vi "Run.vi"(8 "error in (no error)":errorcluster, 11 "App in":refnum<class "App.lvclass">) -> (0 "error out":errorcluster, 3 "App out":refnum<class "App.lvclass">)   [LabVIEW 2022 SP3, in "VMR-Deck.lvlib" / "App.lvclass"]
uses:
  App.lvclass
  App.lvclass/App.ctl
  WebServer/WebServer.lvclass
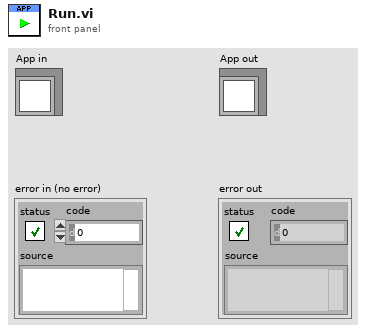
[diagram p1: front panel]
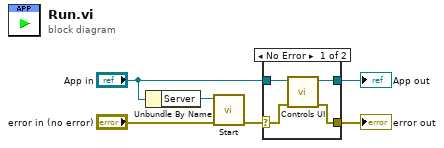
[diagram p0: block diagram]
diagram:
  n1 = Unbundle By Name("App in") -> ("Server"=w4:refnum<class "WebServer.lvclass">)
  n2 = call "Start.vi"("error in (no error)"="error in (no error)", "WebServer in"=w4) -> ("error out"=w2:errorcluster)  [unwired: 8 in, 1 out]
  n3 = case shown="No Error" w2 {
    selector: w2 -> [w8 w12]
    tunnel: [w10 w12] -> w6
    tunnel: [w9 w11] -> w5
    tunnel: "App in" -> [w7 w11]
    frame No Error {
      n4 = call "Controls UI.vi"("error in (no error)"=w8, "App in"=w7) -> ("error out"=w10:errorcluster, "App out"=w9:refnum<class "App.lvclass">)  [unwired: 8 in]
    }
    frame Error {
    }
  }
  "error out" <- w6
  "App out" <- w5
